vi "00T_CreateLOGfile.vi"(11 "LOG file":path) -> (3 "refnum out":refnum<file>)   [LabVIEW 2013]
uses:
  <vilib>/Utility/error.llb/whitespace.ctl
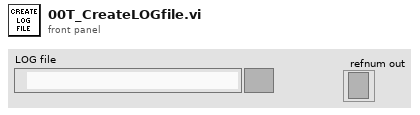
[diagram p1: front panel]
types:
  T1 = typedef "whitespace.ctl" = u16
  T2 = enum16{"open", "replace", "create", "open or create", "replace or create", "replace or create with confirmation"}
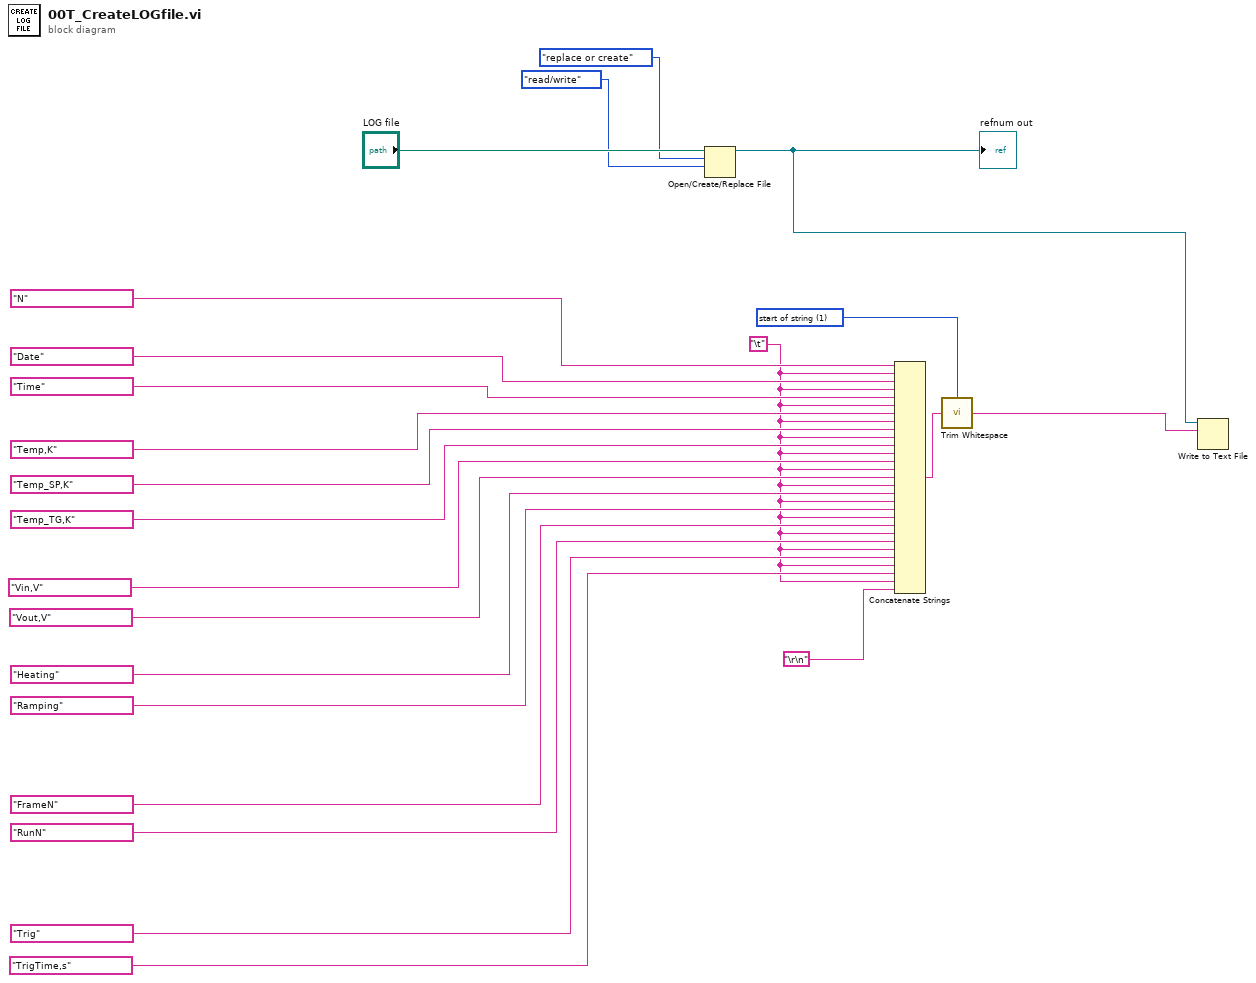
[diagram p0: block diagram]
diagram:
  w2 = "\t"
  w19 = T1 1 items=["both", "start of string", "end of string"] ("location (both)")
  n1 = Open/Create/Replace File(file path (use dialog)="LOG file", operation (0:open)=T2."replace or create", access (0:read/write)=enum16{"read/write", "read-only", "write-only"}."read/write") -> (refnum out=w5:refnum<file>)  [unwired: 3 in, 2 out]
  "refnum out" <- w5
  n2 = Concatenate Strings("N" ("string"), w2, "Date" ("string"), w2, "Time" ("string"), w2, "Temp,K" ("string"), w2, "Temp_SP,K" ("string"), w2, "Temp_TG,K" ("string"), w2, "Vin,V" ("string"), w2, "Vout,V" ("string"), w2, "Heating" ("string"), w2, "Ramping" ("string"), w2, "FrameN" ("string"), w2, "RunN" ("string"), w2, "Trig" ("string"), w2, "TrigTime,s" ("string"), w2, "\r\n") -> (w20:string)
  n3 = call <vilib>:"Trim Whitespace.vi"("string"=w20, "location (both)"=w19) -> ("trimmed string"=w4:string)
  n4 = Write to Text File(file (use dialog)=w5, text=w4) -> ()  [unwired: 2 in, 3 out]
